vi "Start Stream.vi"(8 "error in (no error)":errorcluster, 11 "Pulse Driver in":refnum<class "Pulse Driver.lvclass">) -> (0 "error out":errorcluster, 3 "Pulse Driver out":refnum<class "Pulse Driver.lvclass">)   [LabVIEW 2019, in "Pulse Driver.lvclass"]
uses:
  Pulse Driver.lvclass
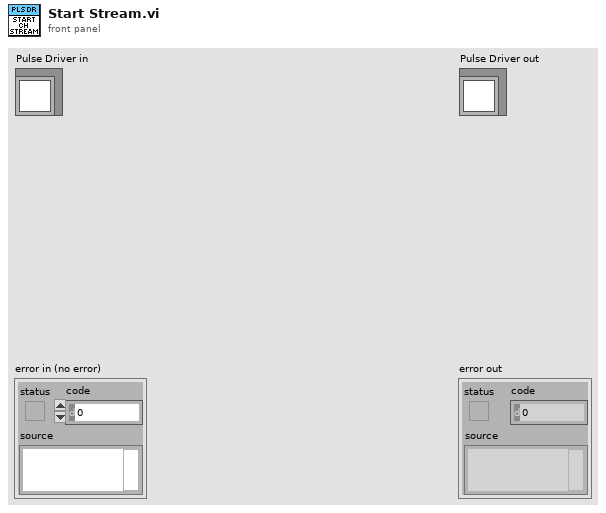
[diagram p1: front panel]
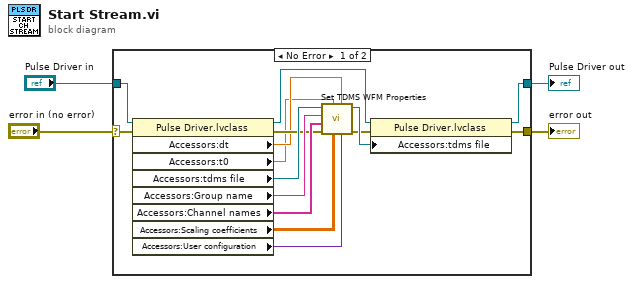
[diagram p0: block diagram]
diagram:
  n1 = case shown="No Error" "error in (no error)" {
    selector: "error in (no error)" -> [w15 w21]
    tunnel: [w16 w21] -> w3
    tunnel: [w17 w20] -> w1
    tunnel: "Pulse Driver in" -> [w19 w20]
    frame No Error {
      n2 = property class="Pulse Driver.lvclass"(reference=w19, error in=w15) -> (reference out=w18:refnum<class "Pulse Driver.lvclass">, error out=w11:errorcluster, "Accessors:dt"=w7:dbl, "Accessors:t0"=w6:dbl, "Accessors:tdms file"=w14:refnum<k34>, "Accessors:Group name"=w13:string, "Accessors:Channel names"=w12:string[], "Accessors:Scaling coefficients"=w8:dbl[][], "Accessors:User configuration"=w5:variant)
      n3 = call "Set TDMS WFM Properties.vi"("Configuration"=w5, "dt"=w7, "Scaling coefficients"=w8, "t0"=w6, "error in (no error)"=w11, "Channel names"=w12, "Group name"=w13, "tdms file"=w14) -> ("error out"=w9:errorcluster, "tdms file out"=w10:refnum<k34>)  [unwired: 2 in]
      n4 = property class="Pulse Driver.lvclass"(reference=w18, error in=w9, "Accessors:tdms file"=w10) -> (reference out=w17:refnum<class "Pulse Driver.lvclass">, error out=w16:errorcluster)
    }
    frame Error {
    }
  }
  "error out" <- w3
  "Pulse Driver out" <- w1
